vi "Add Child Items to Tree.vi"(8 "error in (no error)":errorcluster, 10 "Malleable VI Type in":refnum<class "Malleable VI Type.lvclass">, 11 "Tree Ref in":refnum<vi>) -> (0 "error out":errorcluster, 2 "Malleable VI Type out":refnum<class "Malleable VI Type.lvclass">, 3 "Tree Ref out":refnum<vi>)   [LabVIEW 2020, in "Peek Window.lvlib" / "Malleable VI Type.lvclass"]
uses:
  Malleable VI Type.lvclass
  Symbols Enum.ctl
  Malleable VI Type.lvclass/Malleable VI Type.ctl
  Standard VI Type/Standard VI Type.lvclass/Standard VI Type.ctl
  Standard VI Type/Read Full Qualified Name.vi
  Implementation VI Type/Implementation VI Type.lvclass
  D:/Code/VI-Peek/source/Peek Window/VI Types/Standard VI Type/Standard VI Type.lvclass
  Peek Window.lvlib
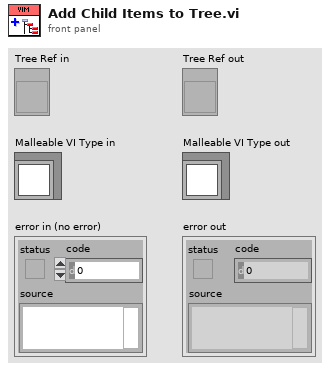
[diagram p1: front panel]
types:
  T1 = typedef "Peek Window.lvlib/Symbols Enum.ctl" = enum16{"<Blank>", "Below Here Glyph", "VI", "Dynamic Dispatch VI", "Malleable VI", "Polymorphic VI", "Missing VI", "Express VI"}
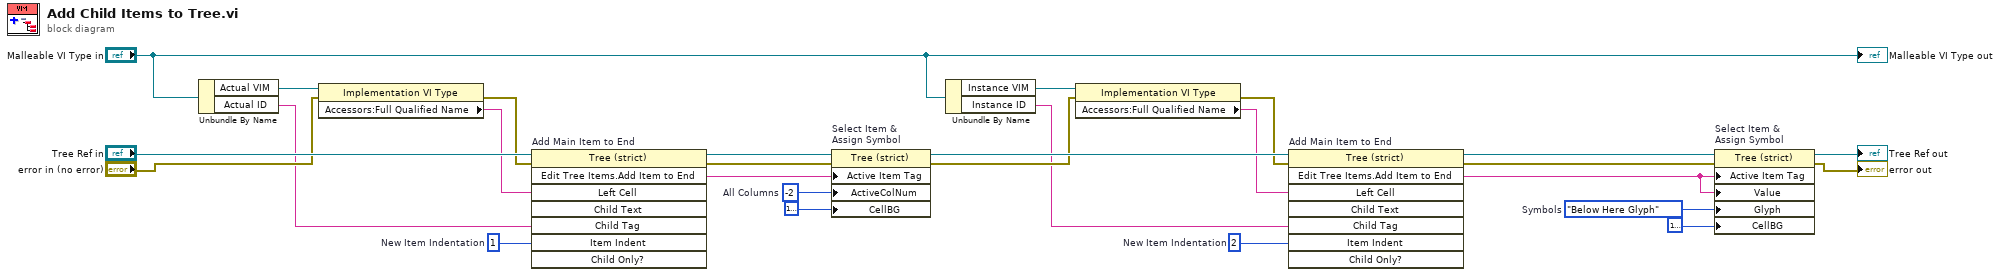
[diagram p0: block diagram]
diagram:
  w2 = -2  # All Columns
  w21 = 2  # New Item Indentation
  w26 = Symbols_Enum."Below Here Glyph"  # Symbols
  w27 = 1  # New Item Indentation
  n1 = Unbundle By Name("Malleable VI Type in") -> ("Actual VIM"=w13:refnum<class "Implementation VI Type.lvclass">, "Actual ID"=w9:string)
  n2 = property class="Implementation VI Type"(reference=w13, error in="error in (no error)") -> (error out=w11:errorcluster, "Accessors:Full Qualified Name"=w10:string)  [unwired: 1 out]
  n3 = invoke on="Add Main Item to End" class="Tree (strict)" method="Edit Tree Items.Add Item to End"(reference="Tree Ref in", error in=w11, "Left Cell"=w10, "Child Tag"=w9, "Item Indent"=w27) -> (reference out=w16:refnum<vi>, error out=w14:errorcluster, "Edit Tree Items:Add Item to End"=w17:string)  [unwired: 3 in, 5 out]
  n4 = property on="Select Item &\nAssign Symbol" class="Tree (strict)"(reference=w16, error in=w14, "Active Item Tag"=w17, "ActiveColNum"=w2, "CellBG"=u32 16777238) -> (reference out=w15:refnum<vi>, error out=w6:errorcluster)
  n5 = Unbundle By Name("Malleable VI Type in") -> ("Instance VIM"=w8:refnum<class "Implementation VI Type.lvclass">, "Instance ID"=w5:string)
  n6 = property class="Implementation VI Type"(reference=w8, error in=w6) -> (error out=w7:errorcluster, "Accessors:Full Qualified Name"=w4:string)  [unwired: 1 out]
  n7 = invoke on="Add Main Item to End" class="Tree (strict)" method="Edit Tree Items.Add Item to End"(reference=w15, error in=w7, "Left Cell"=w4, "Child Tag"=w5, "Item Indent"=w21) -> (reference out=w20:refnum<vi>, error out=w19:errorcluster, "Edit Tree Items:Add Item to End"=w1:string)  [unwired: 3 in, 5 out]
  n8 = property on="Select Item &\nAssign Symbol" class="Tree (strict)"(reference=w20, error in=w19, "Active Item Tag"=w1, "Value"=w1, "Glyph"=w26, "CellBG"=u32 16777238) -> (reference out=→"Tree Ref out":refnum<vi>, error out=→"error out":errorcluster)
  "Malleable VI Type out" <- "Malleable VI Type in"
